vi "Integrate channel in file.vi"(4 "Buffer size":i64=100000, 6 "Offset duration":dbl=0.0095, 7 "group name in":string="Untitled", 8 "Error In":errorcluster, 10 "Integration settings":T1={"Channel"="", "Output name"="", "Factor"=1.0}, 11 "File Path Control":path) -> (0 "Error Out":errorcluster, 2 "Min max":cluster{"Max":dbl, "Min":dbl}, 3 "File Path out":path)   [LabVIEW 2015]
uses:
  <vilib>/Waveform/WDTOps.llb/WDT Number of Waveform Samples DBL.vi
  PulsedMagnetDAQLib/Controls/Integrate channel.ctl
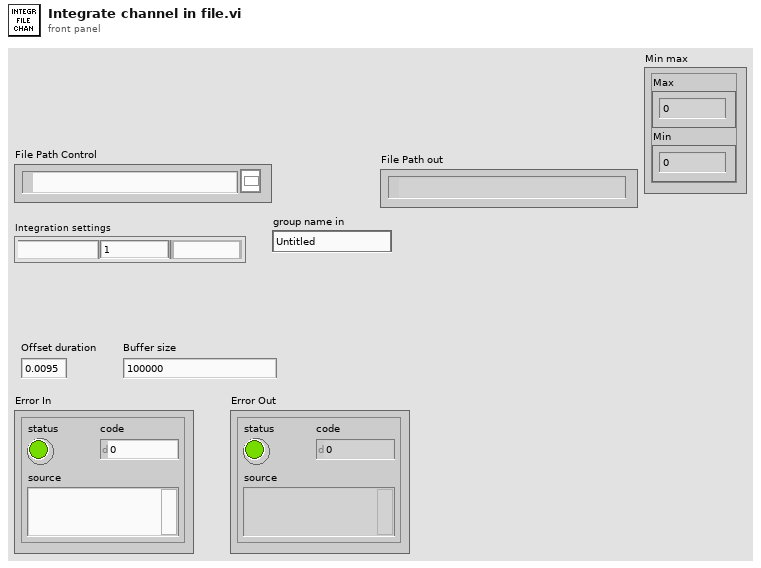
[diagram p1: front panel]
types:
  T1 = typedef "Integrate channel.ctl" = cluster{"Channel":string, "Output name":string, "Factor":dbl}
  T2 = enum16{"open", "open or create", "create or replace", "create", "open (read-only)"}
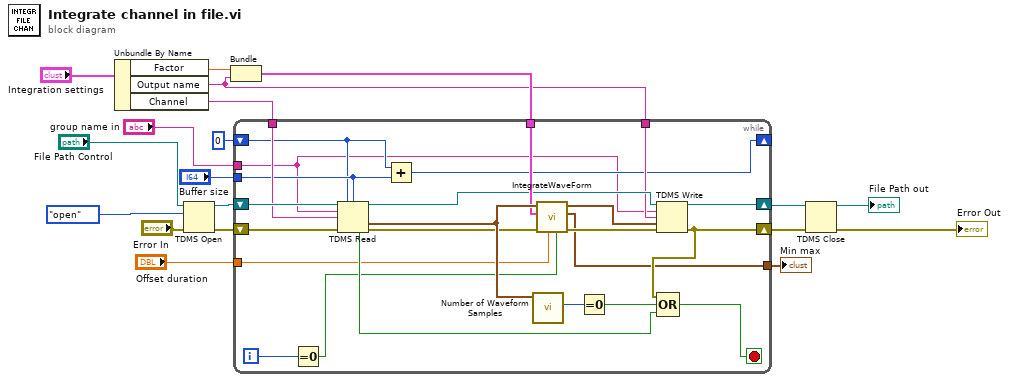
[diagram p0: block diagram]
diagram:
  n1 = Unbundle By Name("Integration settings") -> ("Factor"=w13:dbl, "Output name"=w11:string, "Channel"=w14:string)
  n2 = TDMS Open(8:"Error In", 10:T2."open" ("operation (0:open)"), 11:"File Path Control") -> (0:w10:errorcluster, 3:w16:refnum<k34>)  [unwired: 4 in]
  n3 = Bundle("Factor"=w13, "Output name"=w11) -> (w12:cluster{"Factor":dbl, "Output name":string})  [unwired: 1 in]
  n4 = while {
    tunnel: w14 -> [w41]
    tunnel: w12 -> [w39]
    tunnel: w11 -> [w37]
    shift-right: [w29] -> w9
    shift-left: w10 -> [w32]
    shift-right: [w30] -> w7
    shift-left: w16 -> [w43]
    tunnel: "Buffer size" -> [w27]
    shift-right: [w26] -> _
    shift-left: i64 0 -> [w25]
    tunnel: "Offset duration" -> [w22]
    tunnel: [w21] -> w2
    tunnel: "group name in" -> [w20]
    i -> [w24]
    stop <- w31 stop-if-true
    n5 = Equal To 0?(x=w24) -> (x = 0?=w23:bool)
    n6 = TDMS Read(0:w43, 1:w25, 2:w27, 5:w20, 7:w41, 11:w32) -> (4:w38:refnum<k34>, 10:w40:waveform(dbl), 14:w28:bool, 15:w35:errorcluster)  [unwired: 2 in, 2 out]
    n7 = Add(x=w25, y=w27) -> (x+y=w26:i64)
    n8 = call-poly <vilib>:"Number of Waveform Samples.vi"("waveform in"=w40) -> ("number of samples"=w42:i32)  [unwired: 8 in, 2 out]
    n9 = call "IntegrateWaveForm.vi"("First chunk?"=w23, "Offset duration"=w22, "error in (no error)"=w35, "Integrate settings"=w39, "Waveform"=w40) -> ("error out"=w34:errorcluster, "Min max"=w21:cluster{"Max":dbl, "Min":dbl}, "Integrated Waveform"=w36:waveform(dbl))  [unwired: 4 in]
    n10 = Equal To 0?(x=w42) -> (x = 0?=w33:bool)
    n11 = TDMS Write(0:w38, 5:w20, 7:w37, 9:w36, 11:w34) -> (4:w30:refnum<k34>, 15:w29:errorcluster)  [unwired: 1 in, 2 out]
    n12 = Compound Arithmetic op=OR(w29, w33, w28) -> (w31:bool)
  }
  "Min max" <- w2
  n13 = TDMS Close(8:w9, 11:w7) -> (0:→"Error Out":errorcluster, 3:→"File Path out":path)
